vi "Newport_PM_USB_Open.vi"(8 "Error In":errorcluster) -> (0 "error out":errorcluster, 1 "OpenDevices":bool, 2 "Output:":string, 3 "new reference":refnum<k24>, 4 "Error":bool)   [LabVIEW 2017]
uses:
  C:/Program Files (x86)/Newport/Newport USB Driver/Bin/UsbDllWrap.dll
  Program Files (x86)/Newport/Newport USB Driver/Bin/UsbDllWrap.dll
panel:
  # "Built upon Newport\nUSB Driver v4.2.2"
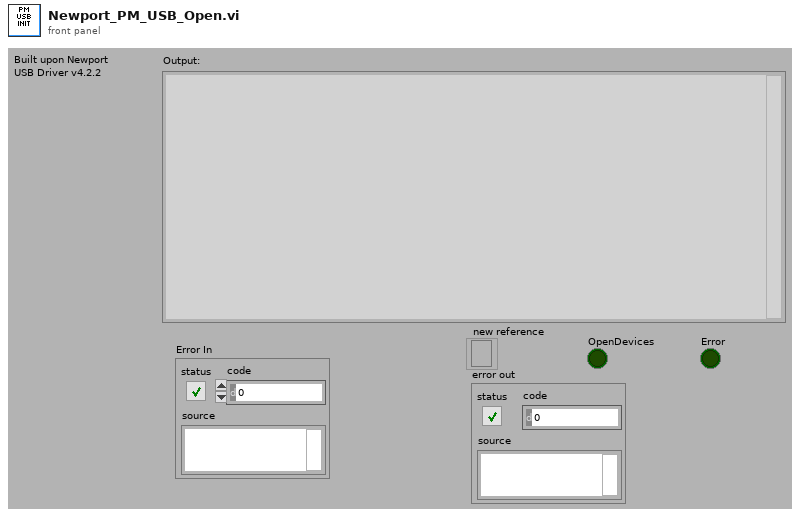
[diagram p1: front panel]
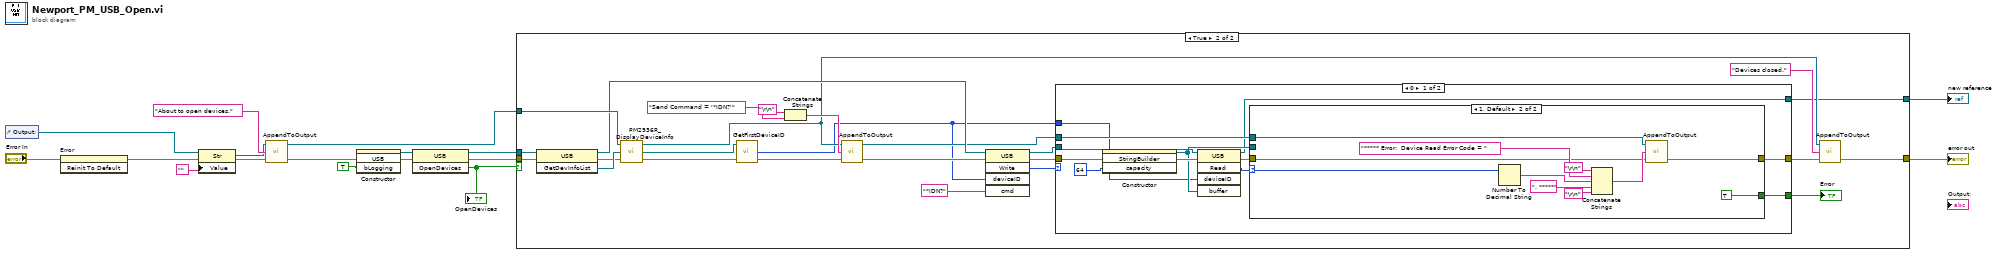
[diagram p0: block diagram]
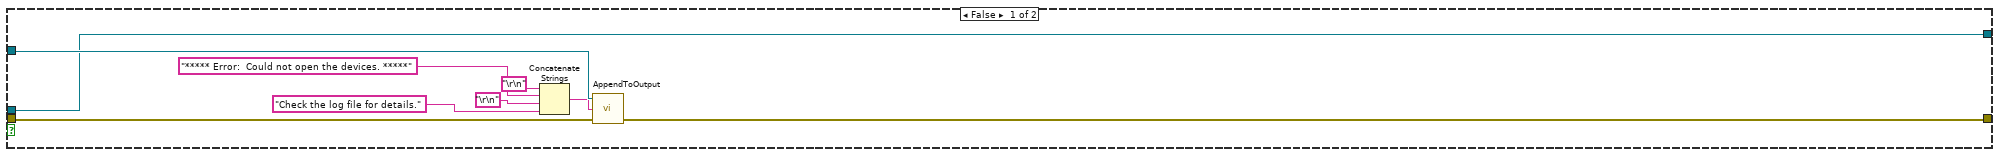
[diagram p2: hidden frame]
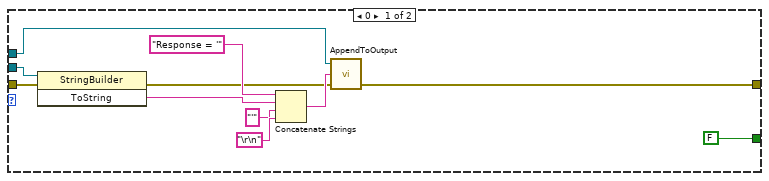
[diagram p3: hidden frame]
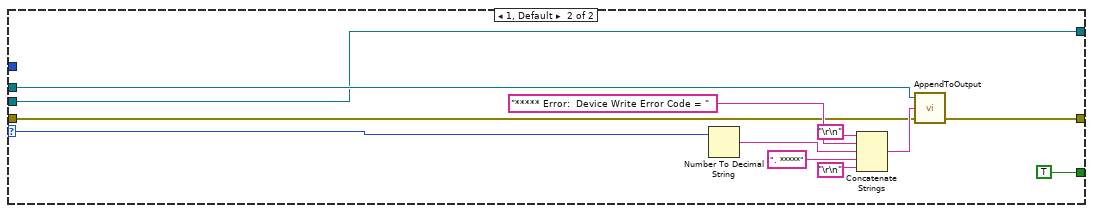
[diagram p4: hidden frame]
diagram:
  n1 = control-ref of="Output:"() -> (w8:refnum<vi>)
  n2 = invoke on="Error" class="Bool (strict)" method="Reinit To Default"(error in="Error In") -> (error out=w4:errorcluster)  [unwired: 2 in, 2 out]
  n3 = property class="Str"(reference=w8, error in=w4, "Value"="") -> (reference out=w5:refnum<vi>, error out=w6:errorcluster)
  n4 = call "AppendToOutput.vi"("error in"=w6, "Input String"="About to open devices.", "Output Refnum In"=w5) -> ("error out"=w15:errorcluster, "Output Refnum Out"=w12:refnum<vi>)  [unwired: 1 in]
  n5 = constructor class="USB"(error in=w15, "bLogging"=TRUE) -> (reference out=w14:refnum<k24>, error out=w11:errorcluster)  [unwired: 2 in, 2 out]
  n6 = invoke class="USB" method="OpenDevices"(reference=w14, error in=w11) -> (reference out=w9:refnum<k24>, error out=w10:errorcluster, "OpenDevices"=w13:bool)  [unwired: 1 in]
  "OpenDevices" <- w13
  n7 = case shown="True" w13 {
    tunnel: w12 -> [w26 w49]
    tunnel: w10 -> [w25 w50]
    tunnel: w9 -> [w18 w51]
    tunnel: [w18 w28] -> w2
    tunnel: [w19 w27] -> w1
    frame False {
      n8 = Concatenate Strings("\r\n", "***** Error:  Could not open the devices. *****", "\r\n", "Check the log file for details.") -> (w21:string)
      n9 = call "AppendToOutput.vi"("error in"=w25, "Input String"=w21, "Output Refnum In"=w26) -> ("error out"=w19:errorcluster)  [unwired: 1 in, 1 out]
    }
    frame True {
      n10 = invoke class="USB" method="GetDevInfoList"(reference=w51, error in=w50) -> (reference out=w42:refnum<k24>, error out=w47:errorcluster, "GetDevInfoList"=w48:refnum<k24>)  [unwired: 1 in]
      n11 = call "PM2936R_DisplayDeviceInfo.vi"("error in"=w47, "DevInfoList In"=w48, "Output Refnum In"=w49) -> ("error out"=w40:errorcluster, "DevInfoList Out"=w39:refnum<k24>, "Output Refnum Out"=w32:refnum<vi>)
      n12 = call "GetFirstDeviceID.vi"("error in"=w40, "DevInfoList In"=w39) -> ("error out"=w38:errorcluster, "Device ID"=w30:i32)  [unwired: 1 in, 1 out]
      n13 = Concatenate Strings("\r\n", "Send Command = '*IDN?'") -> (w44:string)
      n14 = call "AppendToOutput.vi"("error in"=w38, "Input String"=w44, "Output Refnum In"=w32) -> ("error out"=w41:errorcluster, "Output Refnum Out"=w34:refnum<vi>)  [unwired: 1 in]
      n15 = invoke class="USB" method="Write"(reference=w42, error in=w41, "deviceID"=w30, "cmd"="*IDN?") -> (reference out=w36:refnum<k24>, error out=w35:errorcluster, "Write"=w37:i32)  [unwired: 1 in, 2 out]
      n16 = case shown="0" w37 {
        selector: w37 -> [_ w92]
        tunnel: w36 -> [w63 w87]
        tunnel: w35 -> [w60 w90]
        tunnel: [w56 w89] -> w31
        tunnel: w34 -> [w55 w88]
        tunnel: w30 -> [w54 _]
        tunnel: [w53 w87] -> w28
        tunnel: [w52 TRUE] -> w29
        frame 0 {
          n17 = constructor class="StringBuilder"(error in=w60, "capacity"=64) -> (reference out=w58:refnum<k24>, error out=w61:errorcluster)  [unwired: 2 in, 2 out]
          n18 = invoke class="USB" method="Read"(reference=w63, error in=w61, "deviceID"=w54, "buffer"=w58) -> (reference out=w53:refnum<k24>, error out=w57:errorcluster, "Read"=w59:i32)  [unwired: 1 in, 2 out]
          n19 = case shown="1, Default" w59 {
            selector: w59 -> [_ w80]
            tunnel: w58 -> [w74 _]
            tunnel: w57 -> [w73 w77]
            tunnel: [w66 w76] -> w56
            tunnel: w55 -> [w65 w78]
            tunnel: [FALSE TRUE] -> w52
            frame 0 {
              n20 = invoke class="StringBuilder" method="ToString"(reference=w74, error in=w73) -> (error out=w67:errorcluster, "ToString"=w70:string)  [unwired: 1 in, 1 out]
              n21 = Concatenate Strings("Response = '", w70, "'", "\r\n") -> (w68:string)
              n22 = call "AppendToOutput.vi"("error in"=w67, "Input String"=w68, "Output Refnum In"=w65) -> ("error out"=w66:errorcluster)  [unwired: 1 in, 1 out]
            }
            frame 1, Default {
              n23 = Number To Decimal String(number=w80) -> (decimal integer string=w85:string)  [unwired: 1 in]
              n24 = Concatenate Strings("\r\n", "***** Error:  Device Read Error Code = ", w85, ". *****", "\r\n") -> (w79:string)
              n25 = call "AppendToOutput.vi"("error in"=w77, "Input String"=w79, "Output Refnum In"=w78) -> ("error out"=w76:errorcluster)  [unwired: 1 in, 1 out]
            }
          }
        }
        frame 1, Default {
          n26 = Number To Decimal String(number=w92) -> (decimal integer string=w93:string)  [unwired: 1 in]
          n27 = Concatenate Strings("\r\n", "***** Error:  Device Write Error Code = ", w93, ". *****", "\r\n") -> (w91:string)
          n28 = call "AppendToOutput.vi"("error in"=w90, "Input String"=w91, "Output Refnum In"=w88) -> ("error out"=w89:errorcluster)  [unwired: 1 in, 1 out]
        }
      }
      "Error" <- w29
      n29 = call "AppendToOutput.vi"("error in"=w31, "Input String"="Devices closed." ("string"), "Output Refnum In"=w32) -> ("error out"=w27:errorcluster)  [unwired: 1 in, 1 out]
    }
  }
  "new reference" <- w2
  "error out" <- w1
